vi "Error Handler - Initialize DAQ.vi"(8 "error in":errorcluster) -> (0 "error out":errorcluster)   [LabVIEW 2021]
doc: "If an error is encountered initializing the data acquisition system, record a custom error code and terminate the application."
uses:
  <vilib>/Utility/error.llb/Error Cluster From Error Code.vi
  <vilib>/ErrorRing/Error Ring.xnode
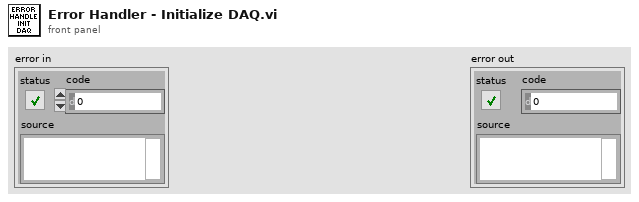
[diagram p1: front panel]
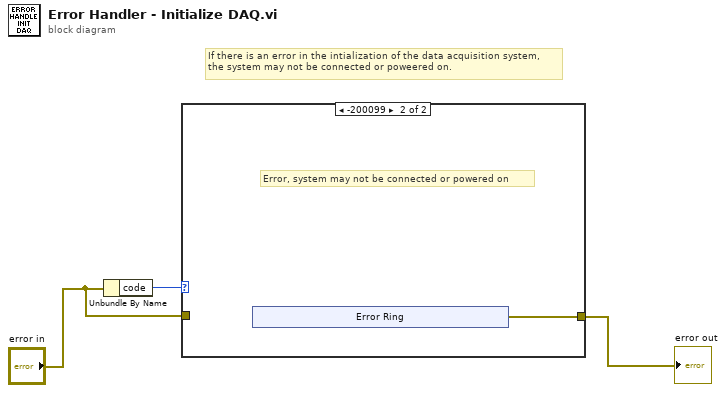
[diagram p0: block diagram]
diagram:
  # "If there is an error in the intialization of the data acquisition system,\nthe system may not be connected or poweered on."
  n1 = Unbundle By Name("error in") -> ("code"=w3:i32)
  n2 = case shown="-200099" w3 {
    tunnel: [w4 w5] -> w2
    tunnel: "error in" -> [w4 _]
    frame 0, Default {
      # "Unhandled error."
    }
    frame -200099 {
      # "Error, system may not be connected or powered on"
      n3 = xnode "Error Ring"() -> ("error out"=w5:errorcluster)
    }
  }
  "error out" <- w2
